vi "Variant_MergeClusters.vi"(10 "New Element(s)":variant, 11 "Original Element(s)":variant) -> (3 "Merged Cluster":variant)   [LabVIEW 2020, in "OpenVariant.lvlib"]
uses:
  OpenVariant.lvlib
  _built_ppls/OpenDescriptor.lvlibp/TypeDescriptor_GetName.vi
  _built_ppls/OpenDescriptor.lvlibp/TypeDescriptor_SetName.vi
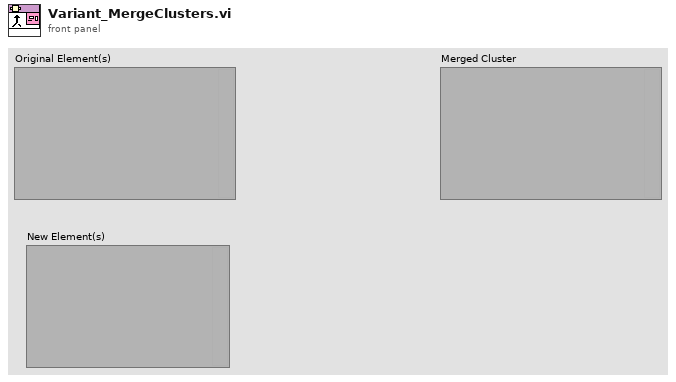
[diagram p1: front panel]
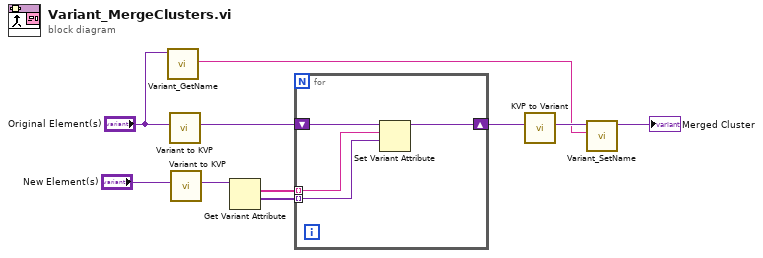
[diagram p0: block diagram]
diagram:
  n1 = call "Variant_GetName.vi"("Variant"="Original Element(s)") -> ("Name"=w1:string)  [unwired: 8 in, 2 out]
  n2 = call "Variant to KVP.vi"("Variant"="Original Element(s)") -> ("KVP Dictionary"=w9:variant)  [unwired: 10 in]
  n3 = call "Variant to KVP.vi"("Variant"="New Element(s)") -> ("KVP Dictionary"=w7:variant)  [unwired: 10 in]
  n4 = Get Variant Attribute(Variant=w7) -> (names=w6:string[], values=w5:variant[])  [unwired: 3 in, 2 out]
  n5 = for {
    shift-right: [w13] -> w8
    shift-left: w9 -> [w14]
    tunnel: w6 -> [w11] mode=indexing
    tunnel: w5 -> [w12] mode=indexing
    n6 = Set Variant Attribute(Variant=w14, name=w11, value=w12) -> (Variant out=w13:variant)  [unwired: 1 in, 2 out]
  }
  n7 = call "KVP to Variant.vi"("KVP"=w8) -> ("Reconstructed Data"=w3:variant)  [unwired: 10 in]
  n8 = call "Variant_SetName.vi"("Name"=w1, "Variant"=w3) -> ("Named Variant"=→"Merged Cluster":variant)  [unwired: 9 in]
